vi "Bifrost.vi"() -> ()   [LabVIEW 2025]
uses:
  <vilib>/OPCUA/NI OPC UA Client.lvlib
  <vilib>/OPCUA/controls/Write Status.ctl
  <vilib>/OPCUA/controls/NodeId.ctl
  <vilib>/OPCUA/client/Multiple Write Double.vi
  <vilib>/OPCUA/client/Connect2.vi
  <vilib>/Utility/error.llb/DialogType.ctl
  <vilib>/numeric/Random Number (Range) DBL.vi
panel:
  out "Waveform Chart":T1(graph)
  out "Temperature (C)":dbl format="%#.2g"
  in  "PI parameters":cluster{"Kp":dbl, "Ti [s]":dbl}={"Kp"=1.3, "Ti [s]"=11.0}
  in  "Reference Value":dbl=50.0
  out "NodeId":string
  in  "Sensor":u16(ring) items=["Simulated", "Air Heater"]
  in  "Sampling intervall":dbl=500.0 caption="Sampling intervall (ms)"
  out "Active":bool
  in  "Cancel Button":bool
  in  "OK Button":bool
  in  "Stop Button":bool
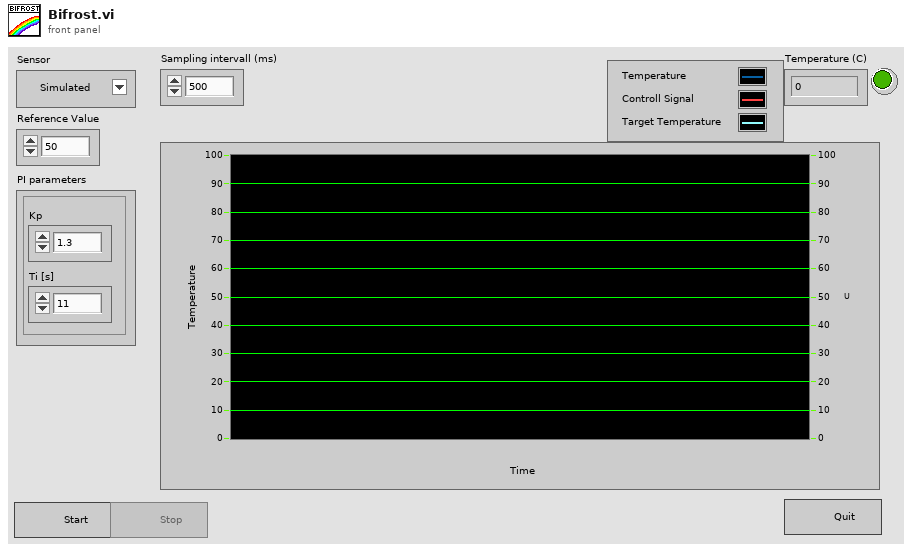
[diagram p1: front panel]
types:
  T1 = cluster{"T_next":dbl, "Control Value (u)":dbl, "Reference Value":dbl}
  T2 = cluster{"T_next":dbl, "Control Value (u)":dbl, "Reference Value":dbl}[]
  T3 = enum8{"Enabled", "Disabled", "Disabled and Grayed Out"}
  T4 = cluster{"message mode":enum16{"None", "Sign", "Sign and Encrypt"}, "security":enum16{"Basic256Sha256", "Aes128Sha256RsaOaep", "Aes256Sha256RsaPss"}}
  T5 = typedef "NodeId.ctl" = string
  T6 = typedef "Write Status.ctl" = u32
  T7 = cluster{"node ID":T5, "value":dbl, "timestamp (current time)":timestamp, "node status":T6}
  T8 = typedef "DialogType.ctl" = u16
  T9 = typedef "OPC UA Client Refnum.ctl" = refnum<k21>
  T10 = cluster{"Temperature [C]":dbl, "Control Value (u)":dbl, "Reference Value":dbl}
  T11 = cluster{"node ID":T5, "value":dbl, "timestamp (current time)":timestamp, "node status":T6}[]
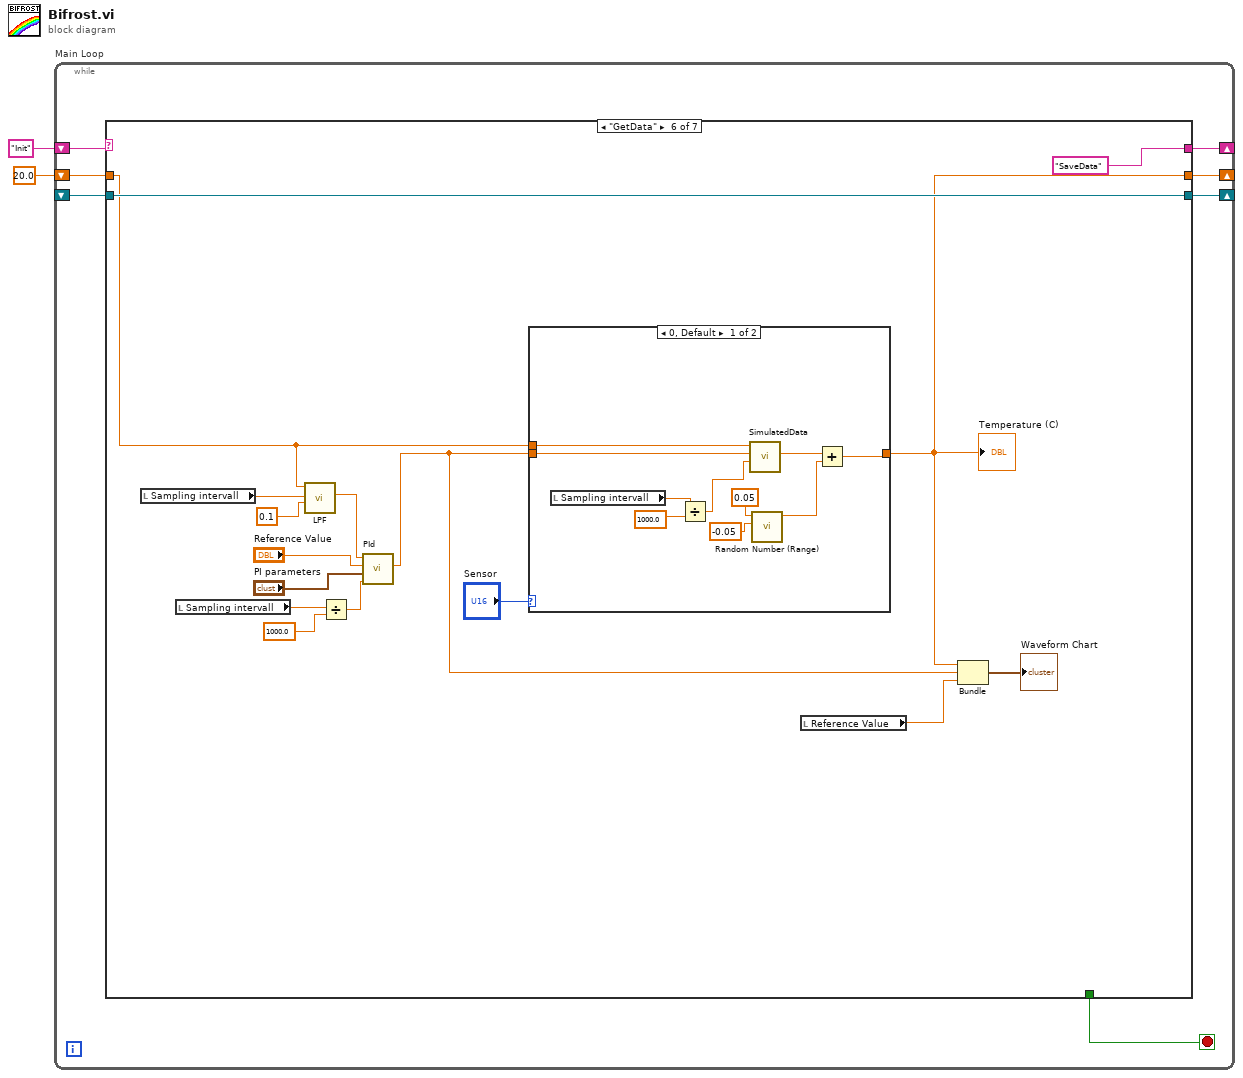
[diagram p0: block diagram]
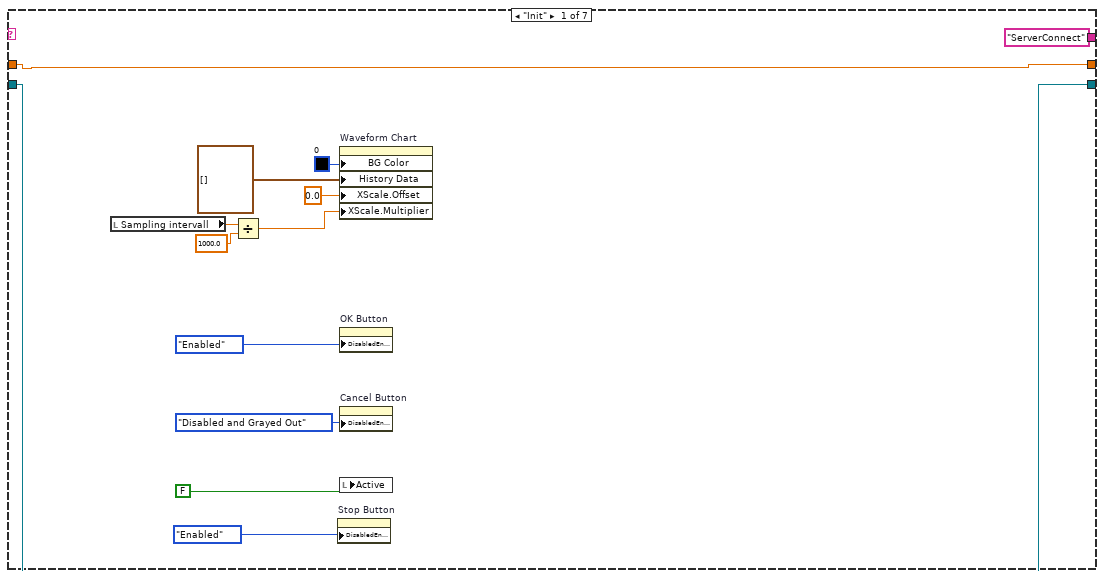
[diagram p2: hidden frame]
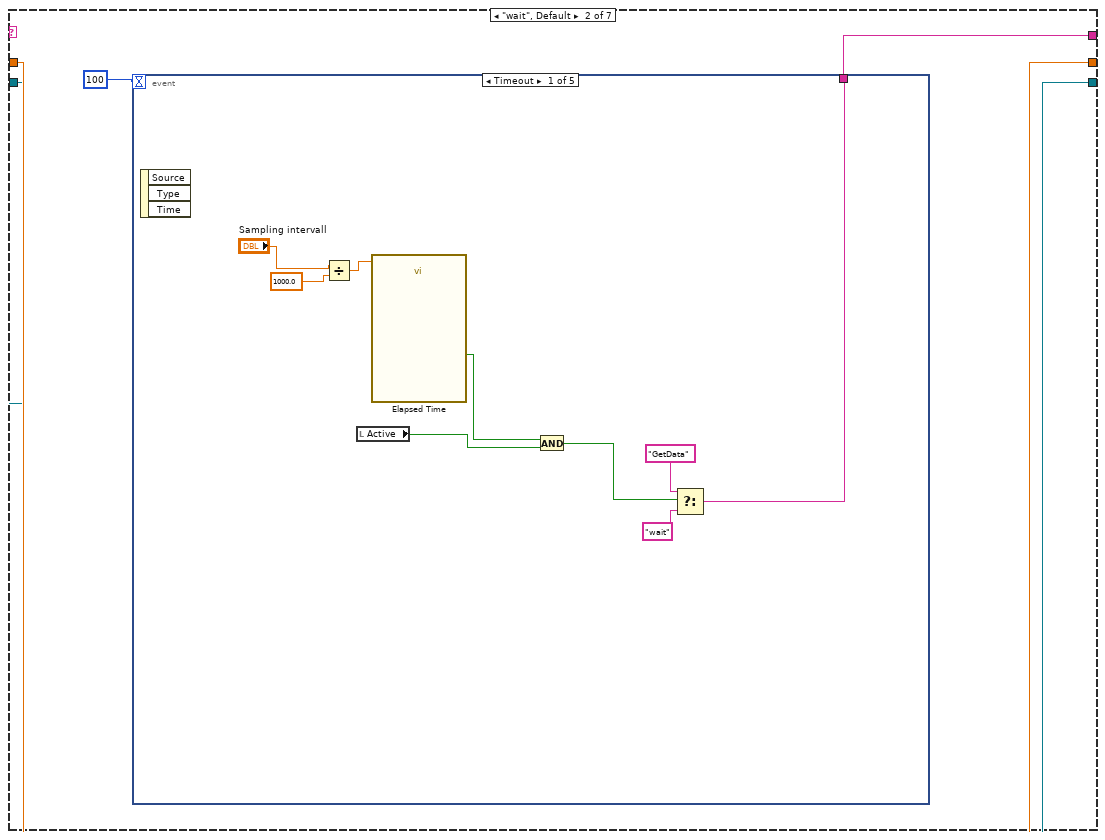
[diagram p3: hidden frame]
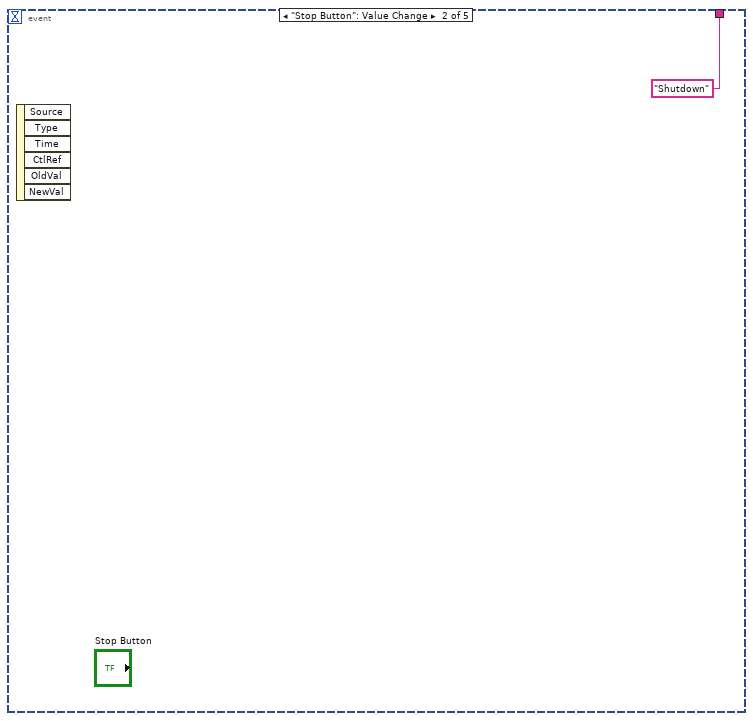
[diagram p4: hidden frame]
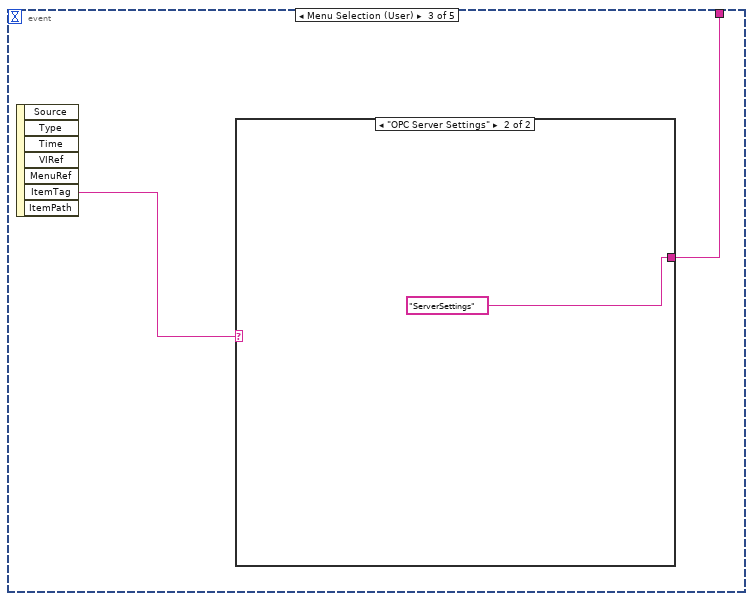
[diagram p5: hidden frame]
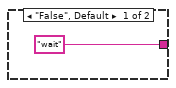
[diagram p6: hidden frame]
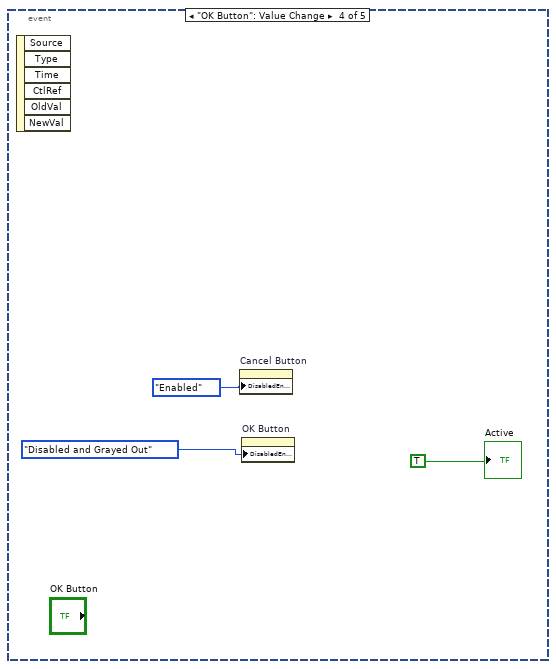
[diagram p7: hidden frame]
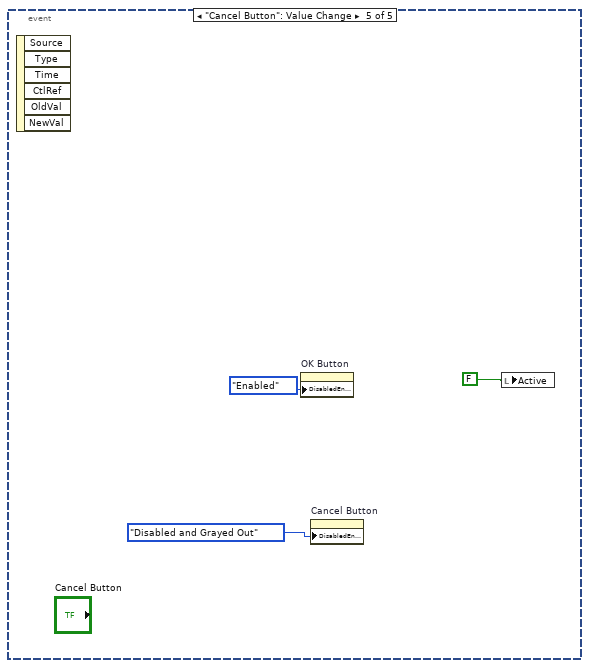
[diagram p8: hidden frame]
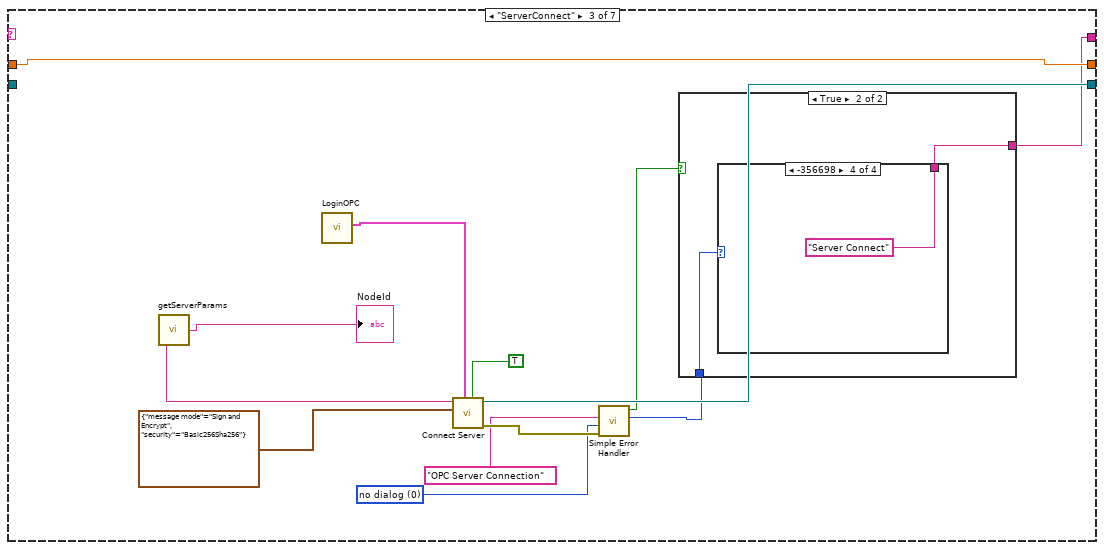
[diagram p9: hidden frame]
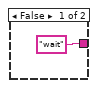
[diagram p10: hidden frame]
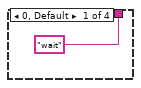
[diagram p11: hidden frame]
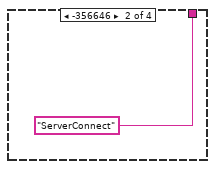
[diagram p12: hidden frame]
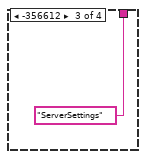
[diagram p13: hidden frame]
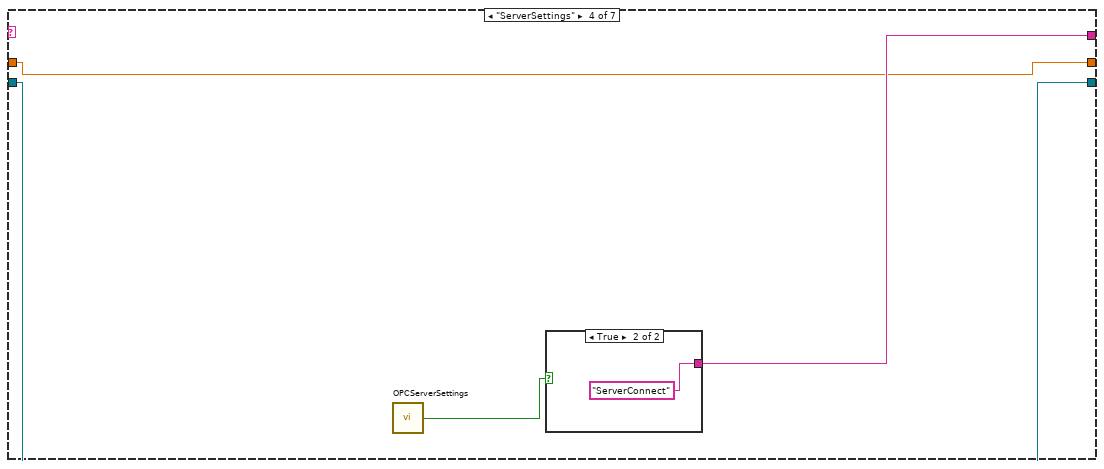
[diagram p14: hidden frame]
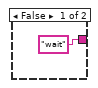
[diagram p15: hidden frame]
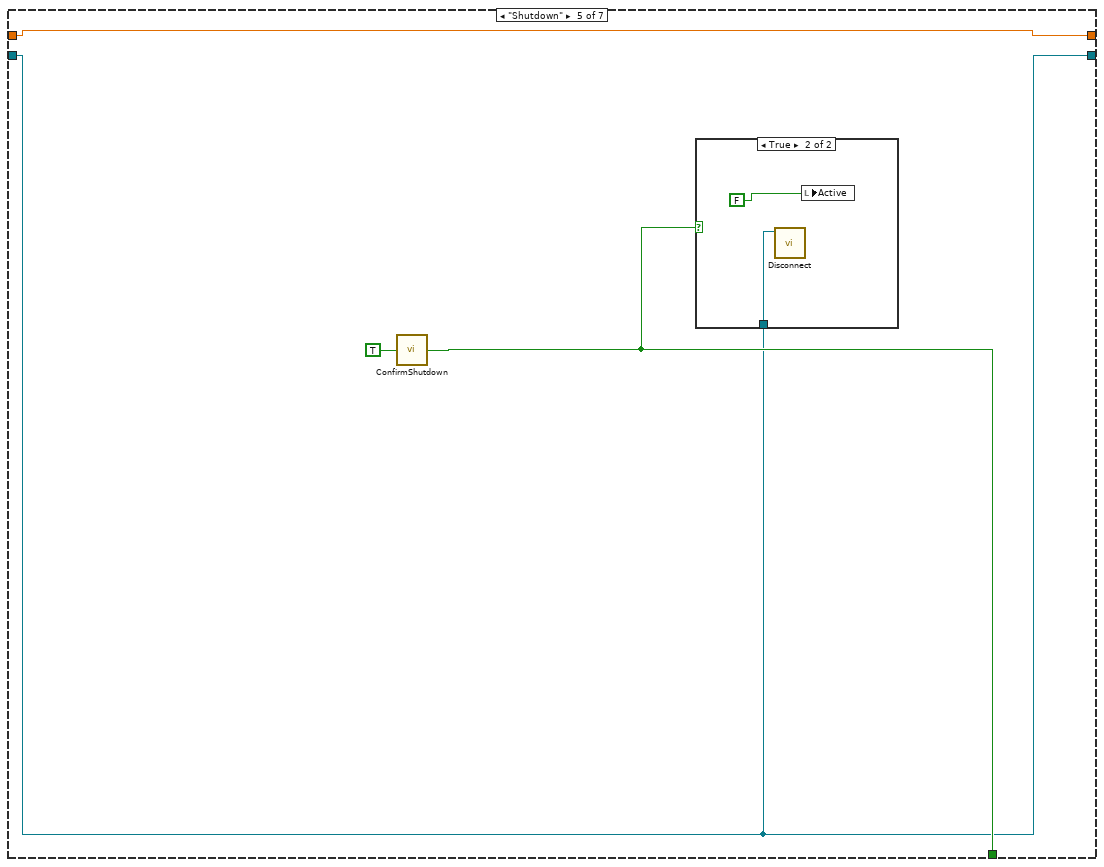
[diagram p16: hidden frame]
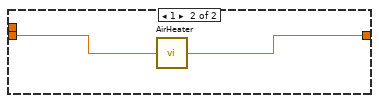
[diagram p18: hidden frame]
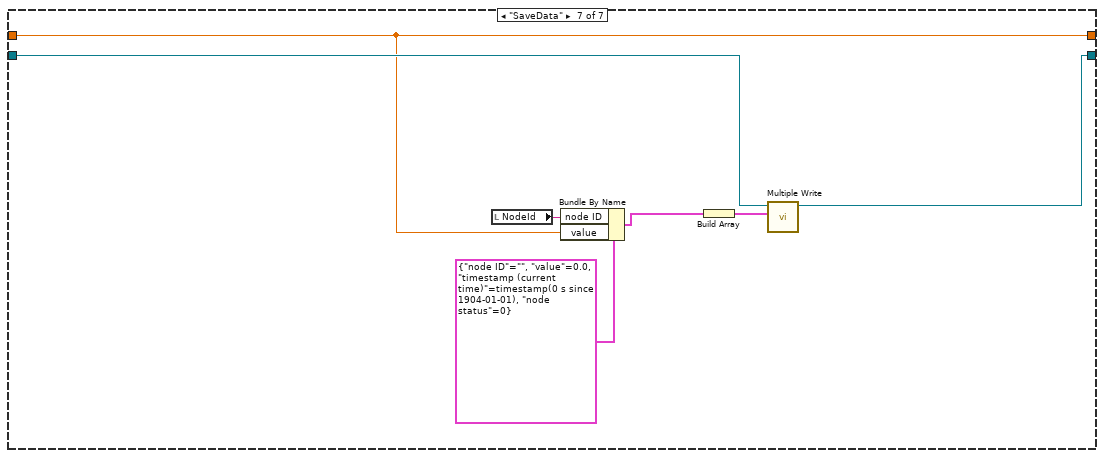
[diagram p19: hidden frame]
diagram:
  n1 = while "Main Loop" {
    shift-right: [w8] -> _
    shift-left: "Init" -> [w9]
    shift-right: [w6] -> _
    shift-left: 20.0 ("T_next") -> [w5]
    shift-right: [w4] -> _
    shift-left: _ -> [w3]
    stop <- w7 stop-if-true
    n2 = case shown="\"GetData\"" w9 {
      tunnel: ["ServerConnect" w25 w48 w69 _ "SaveData" _] -> w8
      tunnel: [_ _ _ _ w74 _ _] -> w7
      tunnel: [w19 w24 w59 w68 w75 w83 w109] -> w6
      tunnel: w5 -> [w19 w24 w59 w68 w75 w81 w109]
      tunnel: [w18 w23 w56 w67 w73 w93 w112] -> w4
      tunnel: w3 -> [w18 w23 _ w67 w73 w93 w113]
      frame "Init" {
        n3 = local read "Sampling intervall"() -> (w12:dbl)
        n4 = Divide(x=w12, y=1000.0) -> (x/y=w10:dbl)
        n5 = property on="Stop Button" class="Bool"("DisabledEnum"=T3."Enabled" ("Disabled")) -> ()  [unwired: 2 in, 2 out]
        n6 = property on="Waveform Chart" class="WFChart (strict)"("BG Color"=u32 0 ("Plot Area:Colors:BG Color"), "History Data"=T2 [], "XScale.Offset"=0.0 ("X Scale.Offset and Multiplier:Offset"), "XScale.Multiplier"=w10) -> ()  [unwired: 2 in, 2 out]
        n7 = property on="OK Button" class="Bool"("DisabledEnum"=T3."Enabled" ("Disabled")) -> ()  [unwired: 2 in, 2 out]
        n8 = property on="Cancel Button" class="Bool"("DisabledEnum"=T3."Disabled and Grayed Out" ("Disabled")) -> ()  [unwired: 2 in, 2 out]
        n9 = local write "Active"(FALSE ("Active")) -> ()
      }
      frame "wait", Default {
        n10 = event shown="[0] Timeout" {
          selector: _ -> [_ _ _ _ _]
          dyn-events: _ -> [_ _ _ _ _]
          timeout: 100 -> [_ _ _ _ _]
          tunnel: [w33 "Shutdown" w37 _ _] -> w25
          event Timeout {
            n11 = event-data() -> ()  [unwired: 1 in, 3 out]
            n12 = Divide(x="Sampling intervall", y=1000.0) -> (x/y=w27:dbl)
            n13 = local read "Active"() -> (w34:bool)
            n14 = call "Elapsed Time"("Time Target (s)"=w27) -> ("Time has Elapsed"=w35:bool)  [unwired: 11 in, 7 out]
            n15 = And(x=w35, y=w34) -> (x .and. y?=w32:bool)
            n16 = Select(t="GetData", s=w32, f="wait") -> (s? t:f=w33:string)
          }
          event "Stop Button": Value Change {
            n17 = event-data() -> ()  [unwired: 1 in, 6 out]
          }
          event Menu Selection (User) {
            n18 = event-data() -> ("ItemTag"=w38:string)  [unwired: 1 in, 6 out]
            n19 = case shown="\"OPC Server Settings\"" w38 {
              tunnel: ["wait" ("f") "ServerSettings" ("f")] -> w37
              frame "False", Default {
              }
              frame "OPC Server Settings" {
              }
            }
          }
          event "OK Button": Value Change {
            n20 = event-data() -> ()  [unwired: 1 in, 6 out]
            n21 = property on="Cancel Button" class="Bool"("DisabledEnum"=T3."Enabled" ("Disabled")) -> ()  [unwired: 2 in, 2 out]
            n22 = property on="OK Button" class="Bool"("DisabledEnum"=T3."Disabled and Grayed Out" ("Disabled")) -> ()  [unwired: 2 in, 2 out]
            "Active" <- TRUE
          }
          event "Cancel Button": Value Change {
            n23 = event-data() -> ()  [unwired: 1 in, 6 out]
            n24 = property on="OK Button" class="Bool"("DisabledEnum"=T3."Enabled" ("Disabled")) -> ()  [unwired: 2 in, 2 out]
            n25 = property on="Cancel Button" class="Bool"("DisabledEnum"=T3."Disabled and Grayed Out" ("Disabled")) -> ()  [unwired: 2 in, 2 out]
            n26 = local write "Active"(FALSE ("Active")) -> ()
          }
        }
      }
      frame "ServerConnect" {
        w50 = T8 0 items=["no dialog", "OK message", "continue or stop message", "OK message + warnings", "continue/stop + warnings"] ("type of dialog (OK msg:1)")
        n27 = call "getServerParams.vi"() -> ("NodeId"=→"NodeId":string, "ServerURL"=w57:string)
        n28 = call "LoginOPC.vi"() -> ("output cluster"=w53:cluster{"Username":string, "Password":string})  [unwired: 11 in]
        n29 = call-poly <vilib>:"Connect Server.vi"("trust any server (F)"=TRUE, "username/password"=w53, "security policy"=T4 {"message mode"=enum."Sign and Encrypt", "security"=enum."Basic256Sha256"}, "server endpoint URL"=w57) -> ("error out"=w52:errorcluster, "OPC UA client refnum out"=w56:T9)  [unwired: 5 in, 1 out]
        n30 = call <vilib>:"Simple Error Handler.vi"("error source (\" \")"="OPC Server Connection" ("error source (\" \")"), "type of dialog (OK msg:1)"=w50, "error in (no error)"=w52) -> ("error?"=w49:bool, "code out"=w47:i32)  [unwired: 2 in, 3 out]
        n31 = case shown="True" w49 {
          tunnel: ["wait" ("f") w62] -> w48
          tunnel: w47 -> [_ w61]
          frame False {
          }
          frame True {
            n32 = case shown="-356698" w61 {
              tunnel: ["wait" ("f") "ServerConnect" ("f") "ServerSettings" ("f") "Server Connect" ("f")] -> w62
              frame 0, Default {
              }
              frame -356646 {
              }
              frame -356612 {
              }
              frame -356698 {
              }
            }
          }
        }
      }
      frame "ServerSettings" {
        n33 = call "OPCServerSettings.vi"() -> ("OK Button 2"=w70:bool)
        n34 = case shown="True" w70 {
          tunnel: ["wait" "ServerConnect"] -> w69
          frame False {
          }
          frame True {
          }
        }
      }
      frame "Shutdown" {
        n35 = call "ConfirmShutdown.vi"("Boolean"=TRUE) -> ("OK Button 2"=w74:bool)
        n36 = case shown="True" w74 {
          tunnel: w73 -> [_ w78]
          frame False {
          }
          frame True {
            n37 = call <vilib>:"Disconnect.vi"("OPC UA client refnum in"=w78) -> ()  [unwired: 10 in, 1 out]
            n38 = local write "Active"(FALSE ("Active")) -> ()
          }
        }
      }
      frame "GetData" {
        n39 = local read "Sampling intervall"() -> (w80:dbl)
        n40 = local read "Sampling intervall"() -> (w90:dbl)
        n41 = call "LPF.vi"("Cutoff freq"=0.1, "Sampling freq"=w80, "x"=w81) -> ("y"=w82:dbl)  [unwired: 8 in]
        n42 = Divide(x=w90, y=1000.0) -> (x/y=w88:dbl)
        n43 = call "PId.vi"("Ts [s]"=w88, "PI Parameters"="PI parameters", "Reference Value"="Reference Value", "Process Value [°C]"=w82) -> ("Control Value (u)"=w85:dbl)  [unwired: 7 in]
        n44 = case shown="0, Default" "Sensor" {
          tunnel: [w99 w105] -> w83
          tunnel: w81 -> [w104 _]
          tunnel: w85 -> [w103 w106]
          frame 0, Default {
            n45 = local read "Sampling intervall"() -> (w102:dbl)
            n46 = Divide(x=w102, y=1000.0) -> (x/y=w100:dbl)
            n47 = call "SimulatedData.vi"("dt"=w100, "u_delayed"=w103, "T(0)"=w104) -> ("T_next"=w98:dbl)  [unwired: 8 in]
            n48 = call-poly <vilib>:"Random Number (Range).vi"("lower bound (0)"=-0.05, "upper bound (100)"=0.05) -> ("number"=w95:dbl)  [unwired: 9 in]
            n49 = Add(x=w98, y=w95) -> (x+y=w99:dbl)
          }
          frame 1 {
            n50 = call "AirHeater.vi"("Controll Signal"=w106) -> ("Temperature [C]"=w105:dbl)
          }
        }
        "Temperature (C)" <- w83
        n51 = local read "Reference Value"() -> (w86:dbl)
        n52 = Bundle "Bundle"("Temperature [C]"=w83, "Control Value (u)"=w85, "Reference Value"=w86) -> (→"Waveform Chart":T10)  [unwired: 1 in]
      }
      frame "SaveData" {
        n53 = local read "NodeId"() -> (w108:string)
        n54 = Bundle By Name "Bundle By Name"(cluster=T7 {"node ID"="", "value"=0.0, "timestamp (current time)"=timestamp(0 s since 1904-01-01), "node status"=0} ("request"), "node ID"=w108, "value"=w109) -> (w107:T7)
        n55 = Build Array(w107) -> (w111:T11)
        n56 = call-poly <vilib>:"Multiple Write.vi"("requests"=w111, "OPC UA client refnum in"=w113) -> ("OPC UA client refnum out"=w112:T9)  [unwired: 6 in, 3 out]
      }
    }
  }
